vi "Get Object Torrent.vi"(8 "error in (no error)":errorcluster, 9 "Bucket":string, 10 "Path":string, 11 "Torrent file path":path=path "") -> (0 "error out":errorcluster, 3 "Torrent file data (RAW)":string)   [LabVIEW 2011, in "LV Interface for Amazon S3.lvlib"]
doc: "This operation <B>returns torrent files from a bucket</B>. BitTorrent can save you bandwidth when you're distributing large files. <B>Note:</B> You can <B>get torrent only for objects</B> that are <B>less than 5 GB</> in size. You must have READ access</B> to the object."
uses:
  LV Interface for Amazon S3.lvlib
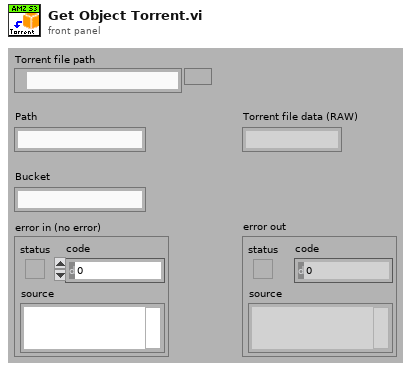
[diagram p1: front panel]
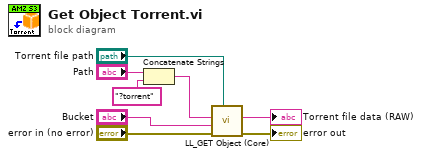
[diagram p0: block diagram]
diagram:
  n1 = Concatenate Strings("Path", "?torrent" ("string")) -> (w3:string)
  n2 = call "LL_GET Object (Core).vi"("output file"="Torrent file path", "error in (no error)"="error in (no error)", "Bucket"="Bucket", "Path and query string"=w3) -> ("error out"=→"error out":errorcluster, "Response body"=→"Torrent file data (RAW)":string)  [unwired: 4 in, 2 out]
